vi "GPIO Command.vi"(10 "Pin(14: NONE)":i32(ring)=14 items=["EXT1", "EXT2", "EXT3", "EXT4", "EXT5", "EXT6", "EXT7", "EXT8", "EXT9", "EXT10", "EXT11", "EXT12", "EXT13", "EXT14", "NONE"]) -> (2 "Command String":string)   [LabVIEW 2023, in "Agilent B2900 Series.lvlib"]
doc: "Parse GPIO pin data into SCIP command string."
uses:
  Agilent B2900 Series.lvlib
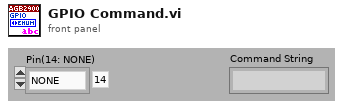
[diagram p1: front panel]
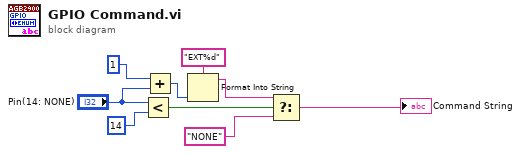
[diagram p0: block diagram]
diagram:
  n1 = Less?(x="Pin(14: NONE)", y=14) -> (x < y?=w3:bool)
  n2 = Add(x=1, y="Pin(14: NONE)") -> (x+y=w7:i32)
  n3 = Format Into String(format string="EXT%d", w7) -> (resulting string=w9:string)  [unwired: 2 in, 1 out]
  n4 = Select(t=w9, s=w3, f="NONE") -> (s? t:f=→"Command String":string)
